vi "Omron Serial FINS-Read Data(Boolean Array).vi"(8 "error in":errorcluster, 10 "Read Setting(Boolean Array)":T1={"I/O Memory Address"=130, "Data Address"=0} {"I/O Memory Address" items=["DM"=130, "CIO"=176, "WR"=177, "HR"=178, "AR"=179, "TIM"=137, "EM"=152]}, 11 "Buffer Data In":T2={"VISA Resource Name"="", "Wait For Read(ms)"=50, "Command Code"=enum."Memory area read", "Command String"="", "Read Bytes"=0, "Response String"=""}) -> (0 "error out":errorcluster, 2 "Data":bool[](array[boolean]), 3 "Buffer Data Out":T2={"VISA Resource Name"="", "Wait For Read(ms)"=50, "Command Code"=enum."Memory area read", "Command String"="", "Read Bytes"=0, "Response String"=""})   [LabVIEW 2016]
uses:
  Data Def/Omron Serial FINS-Buffer Data.ctl
  Data Def/Omron Serial FINS-Command Code.ctl
  Data Def/Omron Serial FINS-FINS Command Frame.ctl
  Data Def/Omron Serial FINS-Memory Area Read Data.ctl
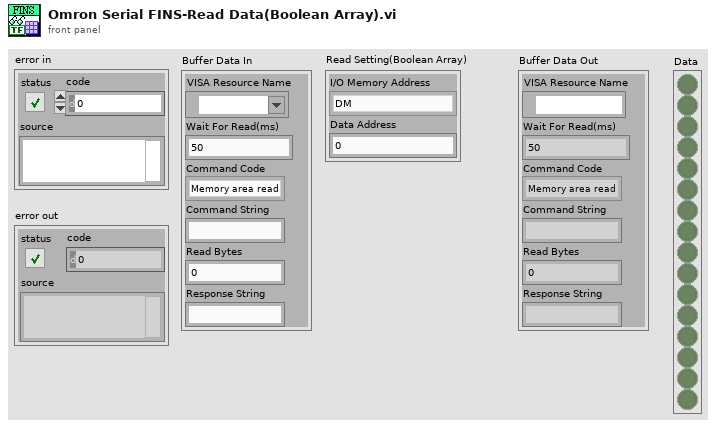
[diagram p1: front panel]
types:
  T1 = cluster{"I/O Memory Address":i32, "Data Address":u32}
  T2 = typedef "Omron Serial FINS-Buffer Data.ctl" = cluster{"VISA Resource Name":refnum<visa-resource-name>, "Wait For Read(ms)":u32, "Command Code":T3, "Command String":string, "Read Bytes":u32, "Response String":string}
  T3 = typedef "Omron Serial FINS-Command Code.ctl" = enum16{"Memory area read", "Memory area write"}
  T4 = typedef "Omron Serial FINS-Memory Area Read Data.ctl" = cluster{"I/O Memory Address":i32, "Beginning Address":u32, "No. Of Items":u32}
  T5 = typedef "Omron Serial FINS-FINS Command Frame.ctl" = cluster{"Unit Number":u8, "Response Wait Time":u8, "Command Code":T3, "Command Data":variant}
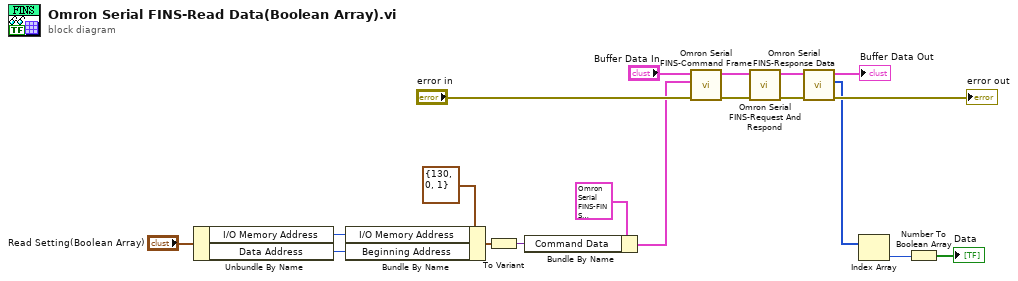
[diagram p0: block diagram]
diagram:
  n1 = Unbundle By Name("Read Setting(Boolean Array)") -> ("I/O Memory Address"=w5:i32, "Data Address"=w4:u32)
  n2 = Bundle By Name(cluster=T4 {"I/O Memory Address"=130, "Beginning Address"=0, "No. Of Items"=1} ("Memory Area Read Data"), "I/O Memory Address"=w5, "Beginning Address"=w4) -> (w8:T4)
  n3 = To Variant(anything=w8) -> (Variant=w17:variant)
  n4 = Bundle By Name(cluster=T5 {"Unit Number"=0, "Response Wait Time"=0, "Command Code"=enum."Memory area read", "Command Data"=variant} ("FINS Command Frame"), "Command Data"=w17) -> (w15:T5)
  n5 = call "Omron Serial FINS-Command Frame.vi"("error in"="error in", "FINS Command Frame"=w15, "Buffer Data In"="Buffer Data In") -> ("error out"=w13:errorcluster, "Buffer Data Out"=w14:T2)  [unwired: 7 in]
  n6 = call "Omron Serial FINS-Request And Respond.vi"("error in"=w13, "Buffer Data In"=w14) -> ("error out"=w11:errorcluster, "Buffer Data Out"=w12:T2)  [unwired: 8 in]
  n7 = call "Omron Serial FINS-Response Data.vi"("error in"=w11, "Buffer Data In"=w12) -> ("error out"=→"error out":errorcluster, "Data"=w3:i16[], "Buffer Data Out"=→"Buffer Data Out":T2)  [unwired: 7 in]
  n8 = Index Array(array=w3) -> (element=w2:i16)  [unwired: 1 in]
  n9 = Number To Boolean Array(number=w2) -> (Boolean array=→"Data":bool[])
